vi "indexing.vi"() -> ()   [LabVIEW 2021]
panel:
  out "String":string
  out "Array":i32[](array[numeric])
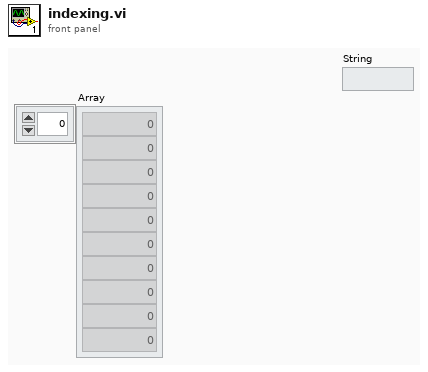
[diagram p1: front panel]
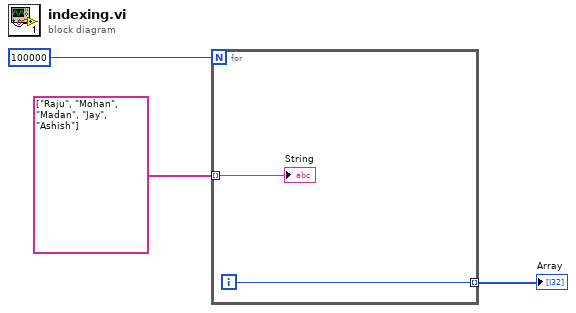
[diagram p0: block diagram]
diagram:
  n1 = for {
    N: 100000 -> [_]
    tunnel: string[] ["Raju", "Mohan", "Madan", "Jay", "Ashish"] -> [w4] mode=indexing
    tunnel: [w5] -> w1 mode=indexing
    i -> [w5]
    "String" <- w4
  }
  "Array" <- w1
